vi "run_cmd.vi"   [LabVIEW 2015, in "lv-bin-plink.lvlib" / "v1.lvlib"]
uses:
  v1.lvlib
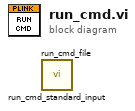
[diagram p0: block diagram]
diagram:
  n1 = call "run_cmd_standard_input.vi"() -> ()  [unwired: 10 in, 2 out]
  n2 = call "run_cmd_file.vi"() -> ()  [unwired: 10 in, 2 out]
